vi "Get Serial Number.vi"(8 "error in (no error)":errorcluster, 11 "nSensorIP":u32) -> (0 "error out":errorcluster, 2 "lpszSerialNum out":string, 3 "function return":i32)   [LabVIEW 2017, in "BonTechWrapperLibrary.lvlib"]
doc: "extern \"C\" BONTECHLIBRARY_API int __stdcall GetSerialNumber(unsigned int nSensorIP, LPTSTR lpszSerialNum);\nextern \"C\" BONTECHLIBRARY_API LPTSTR __stdcall GetSerialNumber(unsigned int nSensorIP, LPTSTR lpszSerialNum);"
uses:
  BonTechWrapperLibrary.lvlib
  BonTechWrapperLibrary.dll
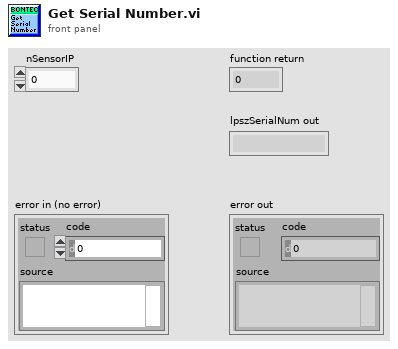
[diagram p1: front panel]
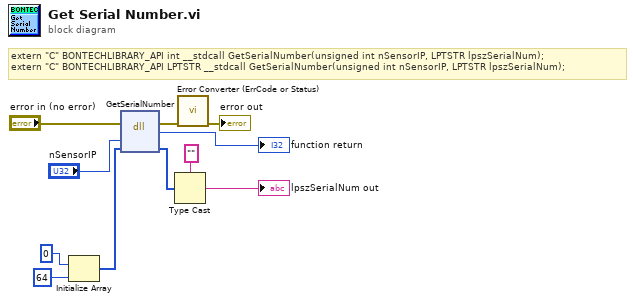
[diagram p0: block diagram]
diagram:
  # "extern \"C\" BONTECHLIBRARY_API int __stdcall GetSerialNumber(unsigned int nSensorIP, LPTSTR lpszSerialNum);\nextern \"C\" BONTECHLIBRARY_API LPTSTR __stdcall GetSerialNumber(unsigned int nSensorIP, LPTSTR lpszSerialNum);"
  n1 = Initialize Array(u8 0 ("Numeric"), 64 ("dimension size")) -> (w5:u8[])
  n2 = dll-call lib="C:/Users/Achuthaperumal/SourceCodes/BonTechWrapperLibrary/BonTechWrapperLibrary/x64/Release/BonTechWrapperLibrary.*" fn="GetSerialNumber"(error in="error in (no error)", "nSensorIP"="nSensorIP", "lpszSerialNum"=w5) -> (error out=w9:errorcluster, "return type"=→"function return":i32, "lpszSerialNum"=w4:u8[])  [unwired: 3 in, 1 out]
  n3 = Type Cast(type="", x=w4) -> (*(type *) &x=→"lpszSerialNum out":string)
  n4 = call "Error Converter (ErrCode or Status).vi"("error in (no error)"=w9) -> ("error out"=→"error out":errorcluster)  [unwired: 10 in]
